vi "EEPROM TestVI.vi"() -> ()   [LabVIEW 2010, in "lib1299.lvlib"]
uses:
  lib1299.lvlib
  <vilib>/Utility/config.llb/Read Key (String).vi
  <userlib>/Common/Queue with Cluster/Enqueue - ClusterBoth.vi
  <vilib>/Utility/config.llb/Write Key (String).vi
  <vilib>/Utility/config.llb/NI_LVConfig.lvlib
panel:
  in  "Close":bool caption="Start"
  out "Written data":string[](array[string])
  out "Connected":bool
  out "Write success":bool
  out "EEPROM Data":string[](array[string])
  in  "Start":bool
  in  "Read EEPROM":bool
  in  "Write EEPROM":bool
  in  "Estyx device name":string
  in  "Firmware file":path
  out "Status box":string
  # "Device Name"
  # "PWB EDGE number and rev"
  # "PCA EDGE number and rev"
  # "BOM EDGE number and rev"
  # "Build Date"
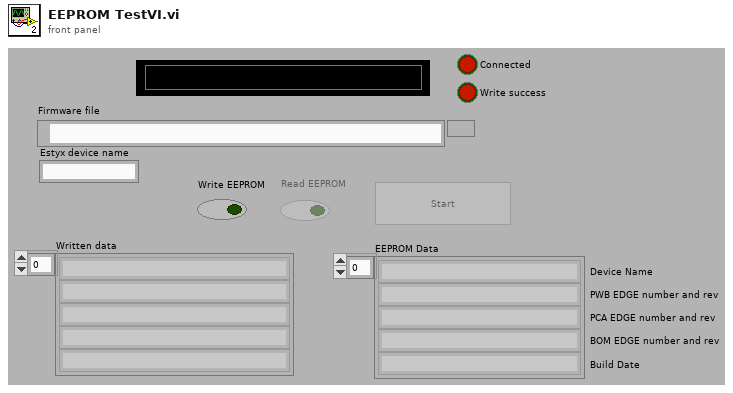
[diagram p1: front panel]
types:
  T1 = enum32{"invalid app kind", "Development System", "Run Time System", "Student Edition", "Embedded LabVIEW", "Evaluation", "Custom"}
  T2 = enum32{"Invalid", "Standard", "Closed", "Hidden", "Minimized", "Maximized"}
  T3 = typedef "TYP_Queue with Cluster Reference.ctl" = refnum<queue>
  T4 = typedef "lib1299.lvlib/EEPROM Tester Info.ctl" = cluster{"client ptr":u32, "connection ptr":u32, "Firmware file":path, "Write VI Reference":refnum<vi>, "Estyx device name":string}
  T5 = typedef "NI_LVConfig.lvlib/Config Data RefNum.ctl" = refnum<k1>
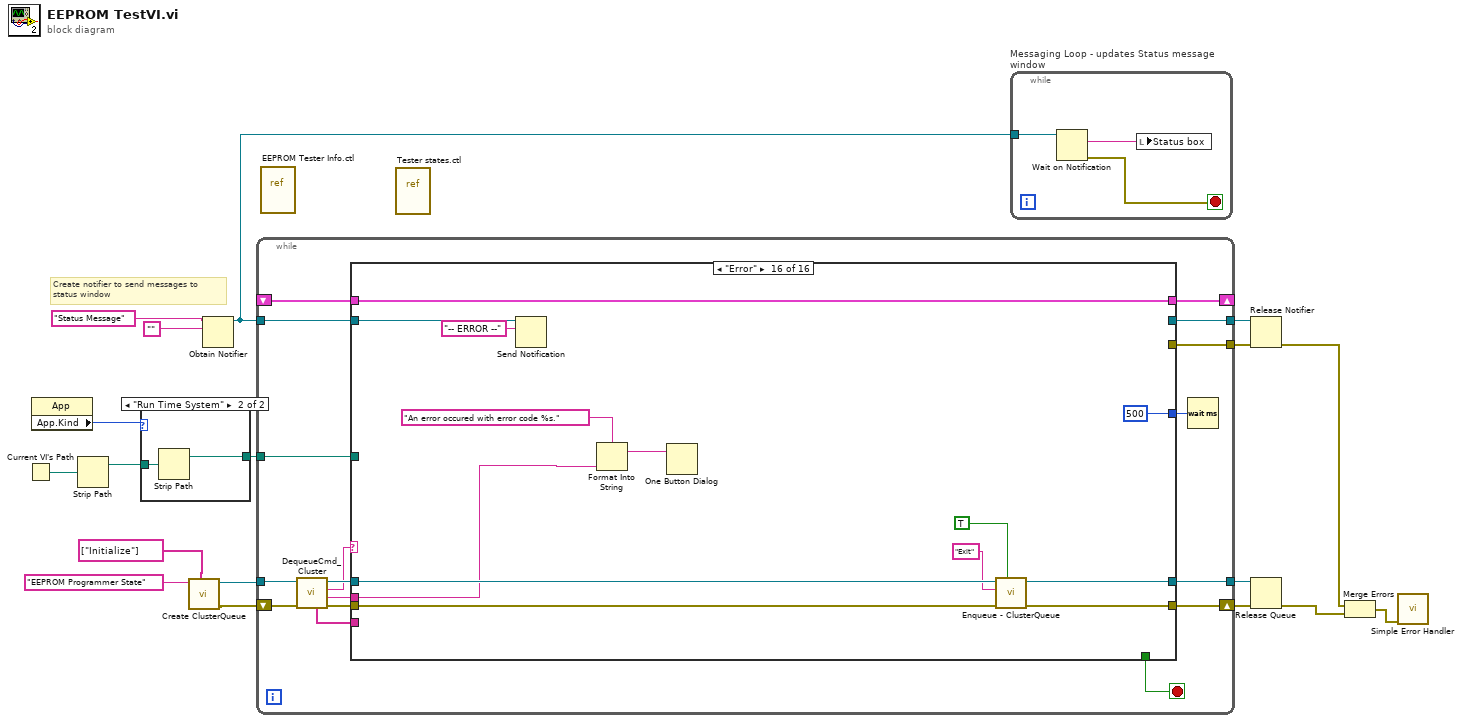
[diagram p0: block diagram]
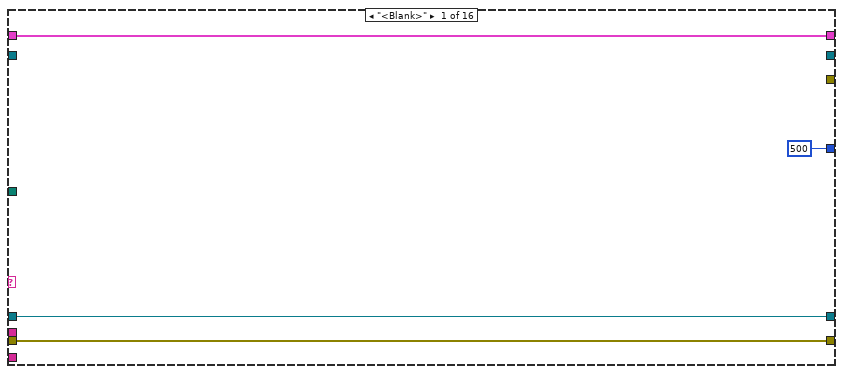
[diagram p3: hidden frame]
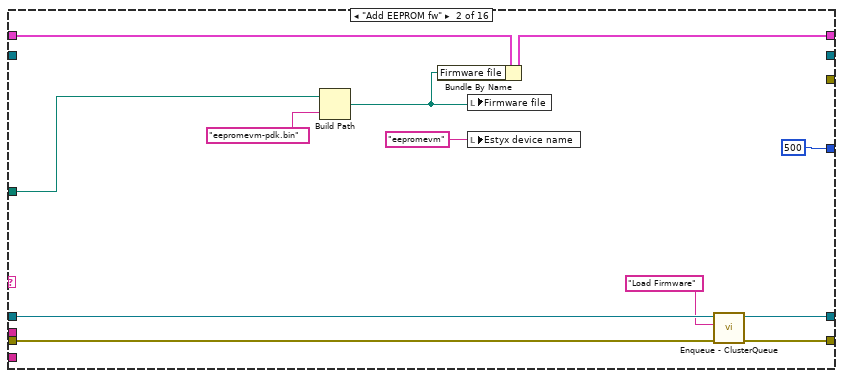
[diagram p4: hidden frame]
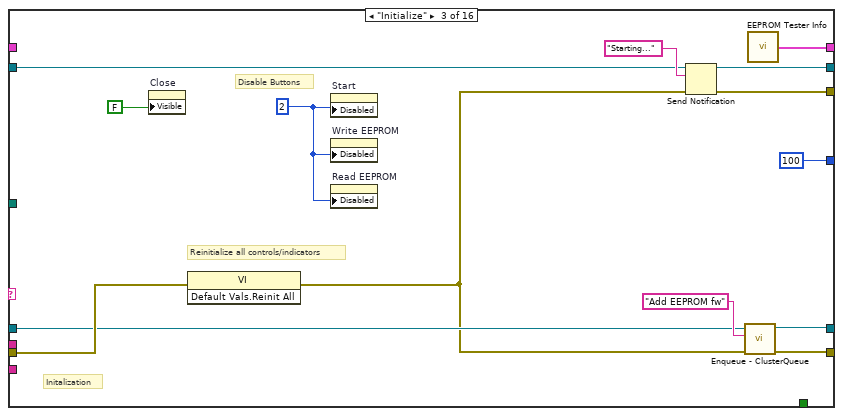
[diagram p5: hidden frame]
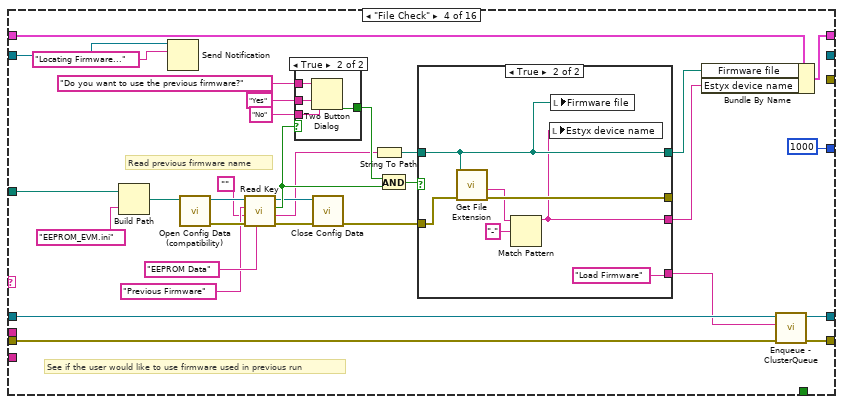
[diagram p6: hidden frame]
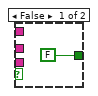
[diagram p7: hidden frame]
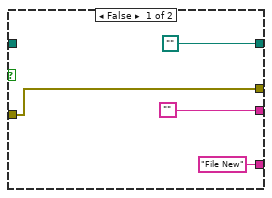
[diagram p8: hidden frame]
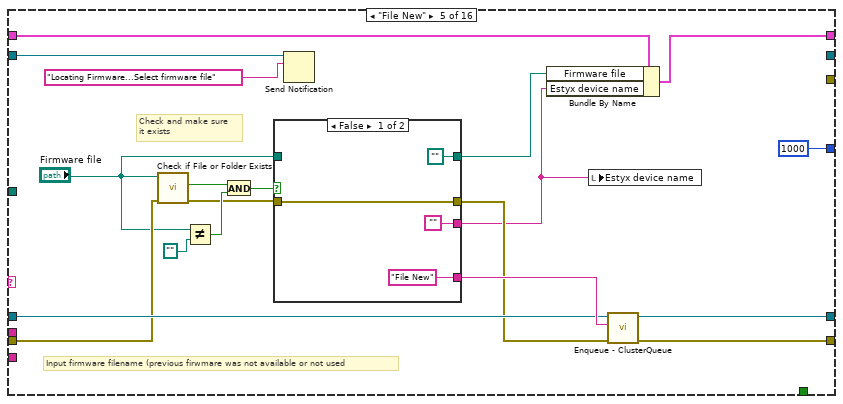
[diagram p9: hidden frame]
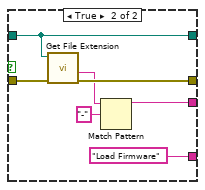
[diagram p10: hidden frame]
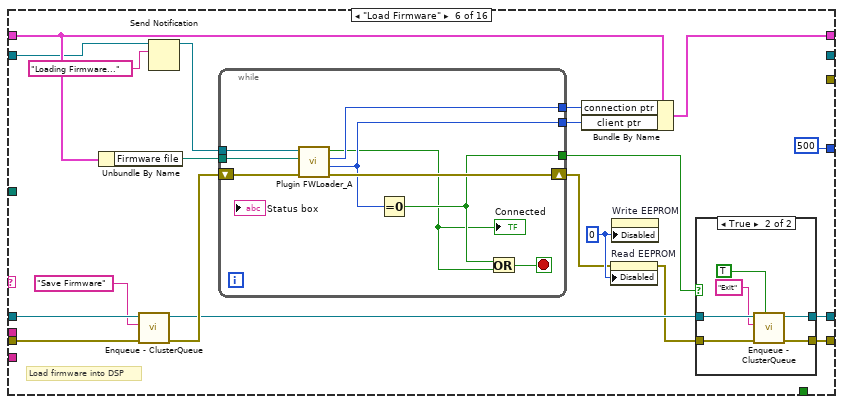
[diagram p11: hidden frame]
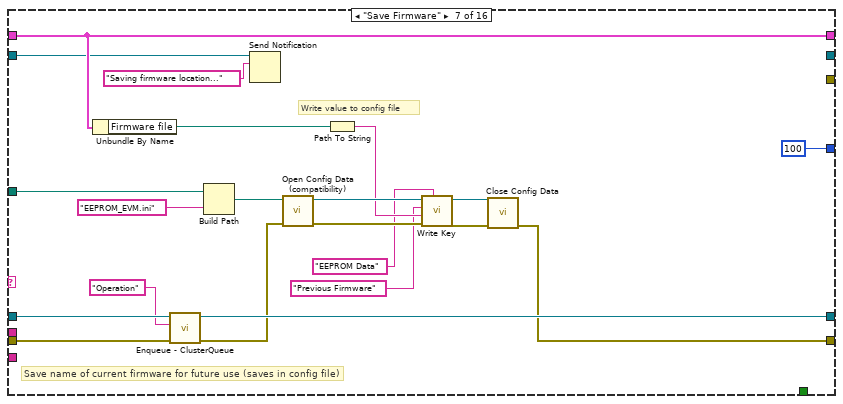
[diagram p13: hidden frame]
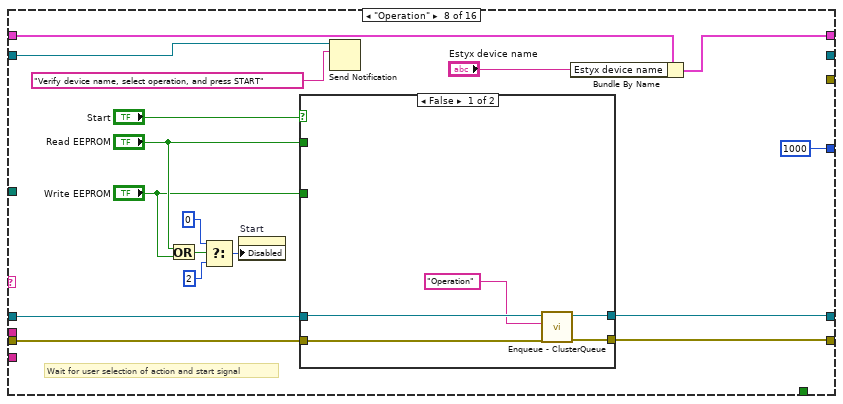
[diagram p14: hidden frame]
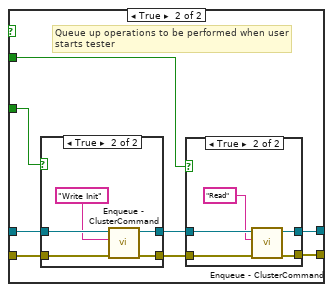
[diagram p15: hidden frame]
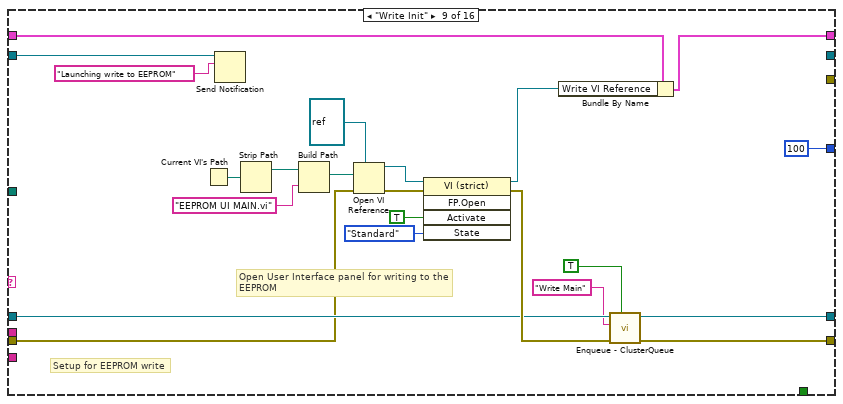
[diagram p18: hidden frame]
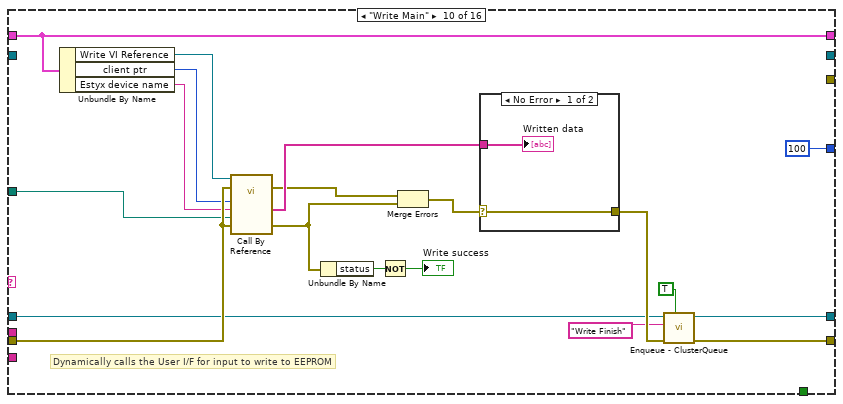
[diagram p19: hidden frame]
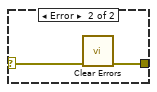
[diagram p20: hidden frame]
diagram:
  # "Create notifier to send messages to\nstatus window"
  n1 = Current VI's Path() -> (path=w15:path)
  n2 = property class="App"() -> ("App.Kind"=w13:T1)  [unwired: 2 in, 2 out]
  n3 = Strip Path(path=w15) -> (stripped path=w16:path)  [unwired: 1 out]
  n4 = case shown="\"Run Time System\"" w13 {
    tunnel: w16 -> [w19 w21]
    tunnel: [w19 w20] -> w14
    frame "Development System", Default {
    }
    frame "Run Time System" {
      n5 = Strip Path(path=w21) -> (stripped path=w20:path)  [unwired: 1 out]
    }
  }
  n6 = call <userlib>:"Create ClusterQueue.vi"("Initial Commands"=string[] ["Initialize"], "Queue Name"="EEPROM Programmer State" ("name (unnamed)")) -> ("error out"=w8:errorcluster, "Queue Out"=w7:refnum<queue>)  [unwired: 8 in]
  n7 = Obtain Notifier(name (unnamed)="Status Message", notification data type="") -> (notifier out=w4:refnum<notifier>)  [unwired: 2 in, 2 out]
  n8 = while {
    shift-right: [w29] -> w17
    shift-left: w8 -> [w38]
    shift-right: [w34] -> _
    shift-left: _ -> [w33]
    tunnel: w14 -> [w28]
    tunnel: w7 -> [w37]
    tunnel: [w30] -> w18
    tunnel: [w24] -> w9
    tunnel: w4 -> [w23]
    tunnel: [w25] -> w10
    stop <- w32 stop-if-true
    n9 = call <userlib>:"DequeueCmd_Cluster.vi"("error in (no error)"=w38, "Queue In"=w37) -> ("error out"=w35:errorcluster, "arg[0]"=w26:string, "command"=w31:string, "queue (dup)"=w36:T3, "arguments"=w22:string[])  [unwired: 4 in, 1 out]
    n10 = case shown="\"Error\"" w31 {
      selector: w31 -> [_ _ _ _ _ _ _ _ _ _ _ _ _ _ w362 _]
      tunnel: w36 -> [w41 w53 w59 w98 w132 w165 w203 w218 w258 w280 w300 w320 w335 w347 w359 w372]
      tunnel: w35 -> [w39 w51 w68 w95 w123 w164 w202 w219 w257 w285 w301 w317 w334 w348 w360 w374]
      tunnel: [w39 w50 w60 w99 w133 w148 w187 w206 w260 w282 w296 w325 w332 w350 w357 w373] -> w29
      tunnel: [w41 w52 w61 w96 w125 w147 w201 w217 w256 w277 w294 w321 w333 w347 w358 w371] -> w30
      tunnel: [w42 w47 w64 w97 w131 w161 w190 w210 w261 w279 w303 w324 w337 w351 w365 w378] -> w34
      tunnel: w33 -> [w42 w48 _ w71 w120 w162 w190 w207 w253 w279 w303 w324 w337 w351 w365 w378]
      tunnel: [_ _ _ _ _ _ _ _ _ _ _ _ _ TRUE _ _] -> w32
      tunnel: w28 -> [_ w43 _ w89 _ _ w191 _ _ w272 _ _ _ _ _ _]
      tunnel: [u32 500 ("milliseconds to wait") u32 500 ("milliseconds to wait") u32 100 ("milliseconds to wait") u32 1000 ("milliseconds to wait") u32 1000 ("milliseconds to wait") u32 500 ("milliseconds to wait") u32 100 ("milliseconds to wait") u32 1000 ("milliseconds to wait") u32 100 ("milliseconds to wait") u32 100 ("milliseconds to wait") u32 500 ("milliseconds to wait") u32 500 ("milliseconds to wait") u32 2000 ("milliseconds to wait") u32 500 ("milliseconds to wait") u32 500 ("milliseconds to wait") u32 500 ("milliseconds to wait")] -> w27
      tunnel: w26 -> [_ _ _ _ _ _ _ _ _ _ _ _ _ _ _ w366]
      tunnel: w23 -> [_ _ w57 w69 w117 w153 w184 w205 w249 _ _ w314 _ w341 w355 w369]
      tunnel: [_ _ w56 _ _ _ _ _ _ _ _ _ _ w339 _ _] -> w25
      tunnel: [_ _ w55 _ _ _ _ _ _ _ _ _ _ w338 _ _] -> w24
      tunnel: w22 -> [_ _ _ _ _ _ _ _ _ _ _ _ _ _ _ _]
      frame "<Blank>" {
      }
      frame "Add EEPROM fw" {
        n11 = Build Path(base path=w43, name or relative path="eepromevm-pdk.bin") -> (appended path=w45:path)
        n12 = Bundle By Name(cluster=w48, "Firmware file"=w45) -> (w47:T4)
        n13 = local write "Firmware file"(w45) -> ()
        n14 = local write "Estyx device name"("eepromevm" ("Estyx device name")) -> ()
        n15 = call-poly <userlib>:"Enqueue - ClusterQueue.vi"("error in (no error)"=w51, "Command"="Load Firmware" ("element"), "Queue with Cluster Reference"=w53) -> ("error out"=w50:errorcluster, "Queue Out (dup)"=w52:T3)  [unwired: 7 in]
      }
      frame "Initialize" {
        w67 = 2
        # "Initalization"
        # "Reinitialize all controls/indicators"
        # "Disable Buttons"
        n16 = property on="Close" class="Bool"("Visible"=FALSE) -> ()  [unwired: 2 in, 2 out]
        n17 = invoke class="VI" method="Default Vals.Reinit All"(error in=w68) -> (error out=w58:errorcluster)  [unwired: 2 in, 2 out]
        n18 = property on="Start" class="Bool"("Disabled"=w67) -> ()  [unwired: 2 in, 2 out]
        n19 = property on="Write EEPROM" class="Bool (strict)"("Disabled"=w67) -> ()  [unwired: 2 in, 2 out]
        n20 = property on="Read EEPROM" class="Bool (strict)"("Disabled"=w67) -> ()  [unwired: 2 in, 2 out]
        n21 = Send Notification(notification="Starting..." ("name (unnamed)"), notifier=w57, error in (no error)=w58) -> (notifier out=w56:refnum<notifier>, error out=w55:errorcluster)
        n22 = call-poly <userlib>:"Enqueue - ClusterQueue.vi"("error in (no error)"=w58, "Command"="Add EEPROM fw" ("element"), "Queue with Cluster Reference"=w59) -> ("error out"=w60:errorcluster, "Queue Out (dup)"=w61:T3)  [unwired: 7 in]
        n23 = call "EEPROM Tester Info.vi"() -> ("EEPROM Tester Info"=w64:T4)  [unwired: 1 in]
      }
      frame "File Check" {
        # "Read previous firmware name"
        # "See if the user would like to use firmware used in previous run"
        n24 = Build Path(base path=w89, name or relative path="EEPROM_EVM.ini") -> (appended path=w87:path)
        n25 = Send Notification(notification="Locating Firmware..." ("Status box"), notifier=w69) -> ()  [unwired: 1 in, 2 out]
        n26 = call <vilib>:"Open Config Data (compatibility).vi"("configuration file path"=w87) -> ("error out"=w92:errorcluster, "refnum"=w93:T5)  [unwired: 8 in, 1 out]
        n27 = call-poly <vilib>:"Read Key.vi"("section"="EEPROM Data", "error in (no error)"=w92, "default value"="", "key"="Previous Firmware" ("section"), "refnum"=w93) -> ("error out"=w78:errorcluster, "value"=w75:string, "found?"=w79:bool, "refnum out"=w76:T5)  [unwired: 3 in]
        n28 = case shown="True" w79 {
          tunnel: "Do you want to use the previous firmware?" ("message") -> [_ w104]
          tunnel: "Yes" ("T button name (\"OK\")") -> [_ w103]
          tunnel: "No" ("F button name (\"Cancel\")") -> [_ w102]
          tunnel: [FALSE ("T button?") w101] -> w80
          frame False {
          }
          frame True {
            n29 = Two Button Dialog(message=w104, 1:w102, 2:w103) -> (T button?=w101:bool)
          }
        }
        n30 = call <vilib>:"Close Config Data.vi"("error in (no error)"=w78, "refnum"=w76) -> ("error out"=w77:errorcluster)  [unwired: 8 in, 1 out]
        n31 = String To Path(string=w75) -> (path=w74:path)
        n32 = And(x=w80, y=w79) -> (x .and. y?=w81:bool)
        n33 = case shown="True" w81 {
          tunnel: ["File New" ("section") "Load Firmware" ("section")] -> w86
          tunnel: [path "" w112] -> w85
          tunnel: w74 -> [_ w112]
          tunnel: [w106 w115] -> _
          tunnel: ["" w110] -> w73
          tunnel: w77 -> [w106 w113]
          frame False {
          }
          frame True {
            n34 = call <vilib>:"Get File Extension.vi"("error in (no error)"=w113, "file"=w112) -> ("error out"=w115:errorcluster, "filename without extension"=w111:string)  [unwired: 6 in, 2 out]
            n35 = Match Pattern(string=w111, regular expression="-") -> (before substring=w110:string)  [unwired: 1 in, 3 out]
            n36 = local write "Estyx device name"(w110) -> ()
            n37 = local write "Firmware file"(w112) -> ()
          }
        }
        n38 = Bundle By Name(cluster=w71, "Firmware file"=w85, "Estyx device name"=w73) -> (w97:T4)
        n39 = call-poly <userlib>:"Enqueue - ClusterQueue.vi"("error in (no error)"=w95, "Command"=w86, "Queue with Cluster Reference"=w98) -> ("error out"=w99:errorcluster, "Queue Out (dup)"=w96:T3)  [unwired: 7 in]
      }
      frame "File New" {
        # "Check and make sure\nit exists"
        # "Input firmware filename (previous firwmare was not available or not used"
        n40 = call <vilib>:"Check if File or Folder Exists.vi"("error in (no error)"=w123, "path"="Firmware file") -> ("error out"=w124:errorcluster, "file or folder exists?"=w128:bool)  [unwired: 7 in, 1 out]
        n41 = Not Equal?(x="Firmware file", y=path "") -> (x != y?=w127:bool)
        n42 = And(x=w128, y=w127) -> (x .and. y?=w129:bool)
        n43 = case shown="False" w129 {
          tunnel: ["File New" ("name (unnamed)") "Load Firmware" ("name (unnamed)")] -> w134
          tunnel: [path "" w145] -> w130
          tunnel: "Firmware file" -> [_ w145]
          tunnel: w124 -> [w137 w144]
          tunnel: [w137 w143] -> w122
          tunnel: ["" w141] -> w121
          frame False {
          }
          frame True {
            n44 = call <vilib>:"Get File Extension.vi"("error in (no error)"=w144, "file"=w145) -> ("error out"=w143:errorcluster, "filename without extension"=w142:string)  [unwired: 6 in, 2 out]
            n45 = Match Pattern(string=w142, regular expression="-") -> (before substring=w141:string)  [unwired: 1 in, 3 out]
          }
        }
        n46 = Send Notification(notification="Locating Firmware...Select firmware file" ("Status box"), notifier=w117) -> ()  [unwired: 1 in, 2 out]
        n47 = Bundle By Name(cluster=w120, "Firmware file"=w130, "Estyx device name"=w121) -> (w131:T4)
        n48 = local write "Estyx device name"(w121) -> ()
        n49 = call-poly <userlib>:"Enqueue - ClusterQueue.vi"("error in (no error)"=w122, "Command"=w134, "Queue with Cluster Reference"=w132) -> ("error out"=w133:errorcluster, "Queue Out (dup)"=w125:T3)  [unwired: 7 in]
      }
      frame "Load Firmware" {
        w158 = u8 0 ("Disabled")
        # "Load firmware into DSP"
        n50 = Unbundle By Name(w162) -> ("Firmware file"=w163:path)
        n51 = call-poly <userlib>:"Enqueue - ClusterQueue.vi"("error in (no error)"=w164, "Command"="Save Firmware" ("name (unnamed)"), "Queue with Cluster Reference"=w165) -> ("error out"=w156:errorcluster, "Queue Out (dup)"=w150:T3)  [unwired: 7 in]
        n52 = Send Notification(notification="Loading Firmware..." ("Status box"), notifier=w153) -> (notifier out=w151:refnum<notifier>)  [unwired: 1 in, 1 out]
        n53 = while {
          tunnel: [w181] -> w160
          tunnel: w163 -> [w182]
          tunnel: [w177] -> w159
          shift-right: [w180] -> w155
          shift-left: w156 -> [w179]
          tunnel: w151 -> [w178]
          tunnel: [w176] -> w146
          stop <- w175 stop-if-true
          n54 = call "Plugin FWLoader_A.vi"("error in (no error)"=w179, "Firmware file"=w182, "Messaging Notifier"=w178) -> ("error out"=w180:errorcluster, "client ptr"=w177:i32, "connection ptr"=w181:i32, "Connected"=w174:bool)  [unwired: 1 in]
          "Connected" <- w174
          n55 = Equal To 0?(x=w177) -> (x = 0?=w176:bool)
          n56 = Or(x=w176, y=w174) -> (x .or. y?=w175:bool)
        }
        n57 = Bundle By Name(cluster=w162, "connection ptr"=w160, "client ptr"=w159) -> (w161:T4)
        n58 = property on="Read EEPROM" class="Bool (strict)"(error in=w155, "Disabled"=w158) -> (error out=w149:errorcluster)  [unwired: 1 in, 1 out]
        n59 = property on="Write EEPROM" class="Bool (strict)"("Disabled"=w158) -> ()  [unwired: 2 in, 2 out]
        n60 = case shown="True" w146 {
          tunnel: w150 -> [w167 w173]
          tunnel: w149 -> [w166 w172]
          tunnel: [w166 w171] -> w148
          tunnel: [w167 w170] -> w147
          frame False {
          }
          frame True {
            n61 = call-poly <userlib>:"Enqueue - ClusterQueue.vi"("At Front?"=TRUE, "error in (no error)"=w172, "Command"="Exit", "Queue with Cluster Reference"=w173) -> ("error out"=w171:errorcluster, "Queue Out (dup)"=w170:T3)  [unwired: 6 in]
          }
        }
      }
      frame "Save Firmware" {
        # "Write value to config file"
        # "Save name of current firmware for future use (saves in config file)"
        n62 = Unbundle By Name(w190) -> ("Firmware file"=w189:path)
        n63 = call-poly <userlib>:"Enqueue - ClusterQueue.vi"("error in (no error)"=w202, "Command"="Operation" ("name (unnamed)"), "Queue with Cluster Reference"=w203) -> ("error out"=w188:errorcluster, "Queue Out (dup)"=w201:T3)  [unwired: 7 in]
        n64 = Build Path(base path=w191, name or relative path="EEPROM_EVM.ini") -> (appended path=w196:path)
        n65 = Send Notification(notification="Saving firmware location...", notifier=w184) -> ()  [unwired: 1 in, 2 out]
        n66 = call <vilib>:"Open Config Data (compatibility).vi"("error in (no error)"=w188, "configuration file path"=w196) -> ("error out"=w200:errorcluster, "refnum"=w199:T5)  [unwired: 7 in, 1 out]
        n67 = Path To String(path=w189) -> (string=w194:string)
        n68 = call-poly <vilib>:"Write Key.vi"("section"="EEPROM Data", "error in (no error)"=w200, "value"=w194, "key"="Previous Firmware" ("section"), "refnum"=w199) -> ("error out"=w197:errorcluster, "refnum out"=w198:T5)  [unwired: 4 in, 1 out]
        n69 = call <vilib>:"Close Config Data.vi"("error in (no error)"=w197, "refnum"=w198) -> ("error out"=w187:errorcluster)  [unwired: 8 in, 1 out]
      }
      frame "Operation" {
        # "Wait for user selection of action and start signal"
        n70 = Or(x="Read EEPROM", y="Write EEPROM") -> (x .or. y?=w213:bool)
        n71 = Select(t=0, s=w213, f=2) -> (s? t:f=w214:i32)
        n72 = property on="Start" class="Bool"("Disabled"=w214) -> ()  [unwired: 2 in, 2 out]
        n73 = case shown="False" "Start" {
          tunnel: w219 -> [w223 w233]
          tunnel: w218 -> [w224 w232]
          tunnel: [w225 w229] -> w206
          tunnel: "Write EEPROM" -> [_ w228]
          tunnel: "Read EEPROM" -> [_ w227]
          tunnel: [w222 w226] -> w217
          frame False {
            n74 = call-poly <userlib>:"Enqueue - ClusterQueue.vi"("error in (no error)"=w223, "Command"="Operation" ("name (unnamed)"), "Queue with Cluster Reference"=w224) -> ("error out"=w225:errorcluster, "Queue Out (dup)"=w222:T3)  [unwired: 7 in]
          }
          frame True {
            # "Queue up operations to be performed when user\nstarts tester"
            n75 = case shown="True" w228 {
              tunnel: w233 -> [w241 w247]
              tunnel: w232 -> [w242 w246]
              tunnel: [w242 w245] -> w231
              tunnel: [w241 w244] -> w230
              frame False {
              }
              frame True {
                n76 = call <userlib>:"Enqueue - ClusterCommand.vi"("error in (no error)"=w247, "Command"="Write Init" ("name (unnamed)"), "Queue with Cluster Reference"=w246) -> ("error out"=w244:errorcluster, "Queue Out (dup)"=w245:T3)  [unwired: 7 in]
              }
            }
            n77 = case shown="True" w227 {
              tunnel: w231 -> [w234 w240]
              tunnel: w230 -> [w235 w239]
              tunnel: [w235 w238] -> w229
              tunnel: [w234 w237] -> w226
              frame False {
              }
              frame True {
                n78 = call <userlib>:"Enqueue - ClusterCommand.vi"("error in (no error)"=w239, "Command"="Read" ("name (unnamed)"), "Queue with Cluster Reference"=w240) -> ("error out"=w238:errorcluster, "Queue Out (dup)"=w237:T3)  [unwired: 7 in]
              }
            }
          }
        }
        n79 = Send Notification(notification="Verify device name, select operation, and press START" ("Status box"), notifier=w205) -> ()  [unwired: 1 in, 2 out]
        n80 = Bundle By Name(cluster=w207, "Estyx device name"="Estyx device name") -> (w210:T4)
      }
      frame "Write Init" {
        # "Open User Interface panel for writing to the\nEEPROM"
        # "Setup for EEPROM write"
        n81 = Current VI's Path() -> (path=w266:path)
        n82 = Send Notification(notification="Launching write to EEPROM" ("Status box"), notifier=w249) -> ()  [unwired: 1 in, 2 out]
        n83 = Strip Path(path=w266) -> (stripped path=w267:path)  [unwired: 1 out]
        n84 = Build Path(base path=w267, name or relative path="EEPROM UI MAIN.vi") -> (appended path=w265:path)
        n85 = Open VI Reference(type specifier VI Refnum (for type only)=refnum<vi> refnum, vi path=w265, error in (no error)=w257) -> (vi reference=w269:refnum<vi>, error out=w268:errorcluster)  [unwired: 3 in]
        n86 = invoke class="VI (strict)" method="FP.Open"(reference=w269, error in=w268, "Activate"=TRUE ("Activate?"), "State"=T2."Standard") -> (reference out=w252:refnum<vi>, error out=w259:errorcluster)  [unwired: 1 in, 3 out]
        n87 = Bundle By Name(cluster=w253, "Write VI Reference"=w252) -> (w261:T4)
        n88 = call-poly <userlib>:"Enqueue - ClusterQueue.vi"("At Front?"=TRUE ("At Front? (F)"), "error in (no error)"=w259, "Command"="Write Main" ("name or relative path"), "Queue with Cluster Reference"=w258) -> ("error out"=w260:errorcluster, "Queue Out (dup)"=w256:T3)  [unwired: 6 in]
      }
      frame "Write Main" {
        # "Dynamically calls the User I/F for input to write to EEPROM"
        n89 = Unbundle By Name(w279) -> ("Write VI Reference"=w283:refnum<vi>, "client ptr"=w284:u32, "Estyx device name"=w278:string)
        n90 = call-by-ref "?"(reference=w283, error in=w285, 4:"error in (no error)"=w285, "Path"=w272, "Estyx device name"=w278, "client ptr"=w284) -> (error out=w286:errorcluster, 0:"error out"=w276:errorcluster, "EDGE/Rev String"=w287:string[])  [unwired: 2 in, 1 out]
        n91 = Unbundle By Name(w276) -> ("status"=w275:bool)
        n92 = Not(x=w275) -> (.not. x?=→"Write success":bool)
        n93 = Merge Errors(w286, w276) -> (w288:errorcluster)
        n94 = case shown="No Error" w288 {
          selector: w288 -> [w290 w291]
          tunnel: w287 -> [w289 _]
          tunnel: [w290 w292] -> w281
          frame No Error {
            "Written data" <- w289
          }
          frame Error {
            n95 = call <vilib>:"Clear Errors.vi"("error in (no error)"=w291) -> ("error out"=w292:errorcluster)  [unwired: 6 in]
          }
        }
        n96 = call-poly <userlib>:"Enqueue - ClusterQueue.vi"("At Front?"=TRUE, "error in (no error)"=w281, "Command"="Write Finish", "Queue with Cluster Reference"=w280) -> ("error out"=w282:errorcluster, "Queue Out (dup)"=w277:T3)  [unwired: 6 in]
      }
      frame "Write Finish" {
        # "Check to see if any more items exist\nin the queue...if not exit"
        # "Close UI for writing"
        # "Complete Write operation"
        n97 = Unbundle By Name(w303) -> ("Write VI Reference"=w302:refnum<vi>)
        n98 = invoke class="VI (strict)" method="FP.Close"(reference=w302, error in=w301) -> (reference out=w304:refnum<vi>, error out=w305:errorcluster)  [unwired: 1 in, 1 out]
        n99 = Close Reference(reference=w304, error in (no error)=w305) -> (error out=w299:errorcluster)
        n100 = Get Queue Status(queue=w300, error in (no error)=w299) -> (queue out=w295:T3, error out=w297:errorcluster, # elements in queue=w298:i32)  [unwired: 1 in, 5 out]
        n101 = case shown="0" w298 {
          tunnel: w297 -> [w308 w312]
          tunnel: [w310 w312] -> w296
          tunnel: w295 -> [w309 w311]
          tunnel: [w307 w311] -> w294
          frame 0 {
            n102 = call <userlib>:"Enqueue - ClusterCommand.vi"("error in (no error)"=w308, "Command"="Exit" ("name (unnamed)"), "Queue with Cluster Reference"=w309) -> ("error out"=w310:errorcluster, "Queue Out (dup)"=w307:T3)  [unwired: 7 in]
          }
          frame Default {
          }
        }
      }
      frame "Read" {
        # "Read the EVM EEPROM"
        n103 = Unbundle By Name(w324) -> ("Estyx device name"=w323:string, "client ptr"=w322:u32)
        n104 = Send Notification(notification="Reading EEPROM" ("Status box"), notifier=w314) -> ()  [unwired: 1 in, 2 out]
        n105 = call "EEPROM Read .vi"("error in (no error)"=w317, "client ptr"=w322, "Estyx device name"=w323) -> ("error out"=w318:errorcluster, "EEPROM data"=→"EEPROM Data":string[])  [unwired: 7 in]
        n106 = call-poly <userlib>:"Enqueue - ClusterQueue.vi"("error in (no error)"=w318, "Command"="Wait" ("name (unnamed)"), "Queue with Cluster Reference"=w320) -> ("error out"=w325:errorcluster, "Queue Out (dup)"=w321:T3)  [unwired: 7 in]
      }
      frame "Wait" {
        w330 = 2
        # "Disable Buttons"
        # "Wait state to allow user to read the EEPROM values read out"
        n107 = property on="Start" class="Bool"("Disabled"=w330) -> ()  [unwired: 2 in, 2 out]
        n108 = property on="Write EEPROM" class="Bool (strict)"("Disabled"=w330) -> ()  [unwired: 2 in, 2 out]
        n109 = property on="Read EEPROM" class="Bool (strict)"("Disabled"=w330) -> ()  [unwired: 2 in, 2 out]
        n110 = property on="Close" class="Bool"("Visible"=TRUE) -> ()  [unwired: 2 in, 2 out]
        n111 = Select(t="Exit" ("name (unnamed)"), s="Close", f="Wait" ("name (unnamed)")) -> (s? t:f=w329:string)
        n112 = call-poly <userlib>:"Enqueue - ClusterQueue.vi"("error in (no error)"=w334, "Command"=w329, "Queue with Cluster Reference"=w335) -> ("error out"=w332:errorcluster, "Queue Out (dup)"=w333:T3)  [unwired: 7 in]
      }
      frame "Exit" {
        # "Exit application if a compiled exe"
        # "Close connections"
        n113 = Unbundle By Name(w351) -> ("client ptr"=w345:u32, "connection ptr"=w344:u32)
        n114 = Send Notification(notification="Exiting" ("Status box"), notifier=w341) -> (notifier out=w339:refnum<notifier>, error out=w338:errorcluster)  [unwired: 1 in]
        n115 = call "lvstyx_close_client.vi"("error in (no error)"=w348, "client ptr"=w345) -> ("error out"=w343:errorcluster)  [unwired: 1 in]
        n116 = call "lvstyx_close_connection.vi"("error in (no error)"=w343, "connection ptr"=w344) -> ("error out"=w350:errorcluster)  [unwired: 1 in]
        n117 = property class="App"() -> ("App.Kind"=w342:T1)  [unwired: 2 in, 2 out]
        n118 = case shown="\"Development System\", Default" w342 {
          frame "Development System", Default {
          }
          frame "Run Time System" {
            n119 = Quit LabVIEW(quit? (T)=TRUE) -> ()
          }
        }
      }
      frame "Developer Error", Default {
        n120 = Send Notification(notification="Invalid command", notifier=w355) -> ()  [unwired: 1 in, 2 out]
        n121 = Format Into String(format string="Developer Error.... \"%s\" is an invalid state.", w362) -> (resulting string=w363:string)  [unwired: 2 in, 1 out]
        n122 = One Button Dialog(message=w363) -> ()  [unwired: 1 in, 1 out]
        n123 = call-poly <userlib>:"Enqueue - ClusterQueue.vi"("At Front? (F)"=TRUE, "error in (no error)"=w360, "Command"="Exit" ("element"), "Queue with Cluster Reference"=w359) -> ("error out"=w357:errorcluster, "Queue Out (dup)"=w358:T3)  [unwired: 6 in]
      }
      frame "Error" {
        n124 = Send Notification(notification="-- ERROR --", notifier=w369) -> ()  [unwired: 1 in, 2 out]
        n125 = Format Into String(format string="An error occured with error code %s.", w366) -> (resulting string=w376:string)  [unwired: 2 in, 1 out]
        n126 = One Button Dialog(message=w376) -> ()  [unwired: 1 in, 1 out]
        n127 = call-poly <userlib>:"Enqueue - ClusterQueue.vi"("At Front?"=TRUE, "error in (no error)"=w374, "Command"="Exit" ("element"), "Queue with Cluster Reference"=w372) -> ("error out"=w373:errorcluster, "Queue Out (dup)"=w371:T3)  [unwired: 6 in]
      }
    }
    n128 = Wait (ms)(milliseconds to wait=w27) -> ()  [unwired: 1 out]
  }
  n129 = vi-ref "EEPROM Tester Info.ctl"() -> ()  [unwired: 1 out]
  n130 = vi-ref "Tester states.ctl"() -> ()  [unwired: 1 out]
  n131 = while "Messaging Loop - updates Status message window" {
    tunnel: w4 -> [w381]
    stop <- w380 stop-if-true
    n132 = Wait on Notification(notifier=w381) -> (notification=w379:string, error out=w380:errorcluster)  [unwired: 3 in, 2 out]
    n133 = local write "Status box"(w379) -> ()
  }
  n134 = Release Notifier(notifier=w10, error in (no error)=w9) -> (error out=w2:errorcluster)  [unwired: 1 in, 2 out]
  n135 = Release Queue(queue=w18, error in (no error)=w17) -> (error out=w3:errorcluster)  [unwired: 1 in, 2 out]
  n136 = Merge Errors(w2, w3) -> (w1:errorcluster)
  n137 = call <vilib>:"Simple Error Handler.vi"("error in (no error)"=w1) -> ()  [unwired: 4 in, 5 out]
